vi "Read Angular Velocity.vi"(8 "error in (no error)":errorcluster, 11 "wheel in":refnum<class "NI_Robotics_Wheel.lvclass">) -> (0 "error out":errorcluster, 1 "failed":bool, 2 "forward angular velocity":dbl, 3 "wheel out":refnum<class "NI_Robotics_Wheel.lvclass">)   [LabVIEW 2017, in "NI_Robotics_Wheel.lvclass"]
uses:
  <vilib>/robotics/Steering/Wheel/NI_Robotics_Wheel.lvclass
  <vilib>/robotics/Steering/Wheel/NI_Robotics_Wheel.lvclass/NI_Robotics_Wheel.ctl
  <vilib>/robotics/Actuation/Motor Communication/Check if Valid.vi
  <vilib>/robotics/Utilities/Generate Error.vi
  <vilib>/robotics/Actuation/Motor Communication/NI_Robotics_Motor Communication.lvclass
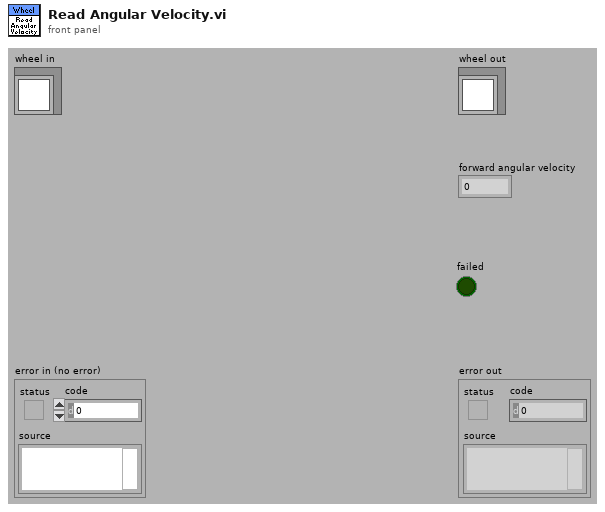
[diagram p1: front panel]
types:
  T1 = typedef "NI_Robotics_Wheel.lvclass/Rotation Direction.ctl" = u16
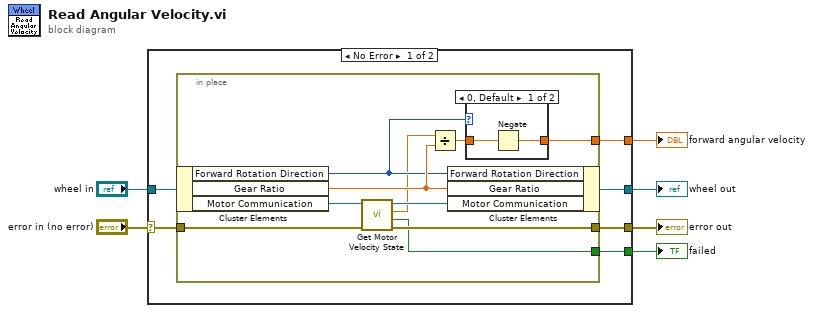
[diagram p0: block diagram]
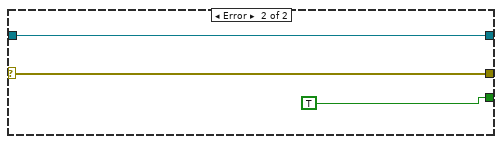
[diagram p3: hidden frame]
diagram:
  n1 = case shown="No Error" "error in (no error)" {
    selector: "error in (no error)" -> [w10 w28]
    tunnel: [w8 w28] -> w5
    tunnel: [w11 w27] -> w3
    tunnel: "wheel in" -> [w12 w27]
    tunnel: [w9 _] -> w2
    tunnel: [w7 TRUE] -> w1
    frame No Error {
      n2 = in-place {
        in-place-border: w10 -> [w15]
        in-place-border: [w20] -> w9
        in-place-border: [w14] -> w8
        in-place-border: [w13] -> w7
        n3 = in-place-cluster #1(w12) -> ("Forward Rotation Direction"=w19:T1, "Gear Ratio"=w22:dbl, "Motor Communication"=w18:refnum<class "NI_Robotics_Motor Communication.lvclass">)
        n4 = call <vilib>:"Get Motor Velocity State.vi"("error in (no error)"=w15, "motor communication in"=w18) -> ("error out"=w14:errorcluster, "failed?"=w13:bool, "velocity"=w16:dbl, "motor communication out"=w17:refnum<class "NI_Robotics_Motor Communication.lvclass">)  [unwired: 6 in]
        n5 = Divide(x=w16, y=w22) -> (x/y=w21:dbl)
        n6 = in-place-cluster #1("Forward Rotation Direction"=w19, "Gear Ratio"=w22, "Motor Communication"=w17) -> (w11:refnum<class "NI_Robotics_Wheel.lvclass">)
        n7 = case shown="0, Default" w19 {
          tunnel: w21 -> [w24 w25]
          tunnel: [w23 w25] -> w20
          frame 0, Default {
            n8 = Negate(x=w24) -> (-x=w23:dbl)
          }
          frame 1 {
          }
        }
      }
    }
    frame Error {
    }
  }
  "error out" <- w5
  "wheel out" <- w3
  "forward angular velocity" <- w2
  "failed" <- w1
